vi "CreateVIActivationVIDesactivation.vi"(8 "error in (no error)":errorcluster, 11 "Menu in":refnum<class "VIActivation.lvclass">) -> (0 "error out":errorcluster, 3 "Menu out":refnum<class "VIActivation.lvclass">)   [LabVIEW 2021, in "VIActivation.lvlib" / "VIActivation.lvclass"]
uses:
  VIActivation.lvclass
  VIActivation.lvclass/VIActivation.ctl
  VIActivationEvents.ctl
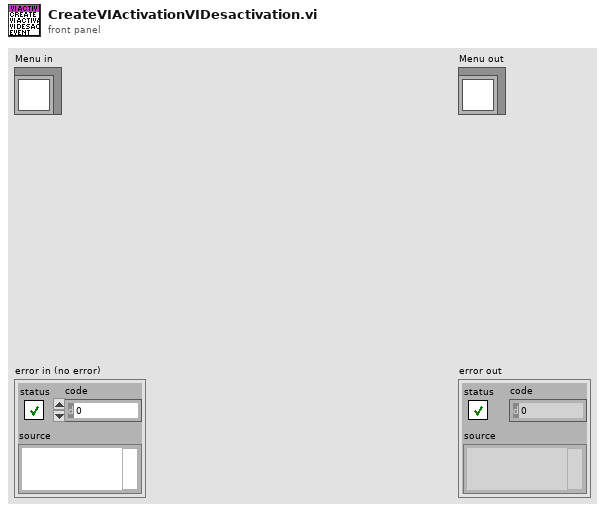
[diagram p1: front panel]
types:
  T1 = typedef "VIActivation.lvlib/VIActivation.lvclass/VIActivationEvents.ctl" = cluster{"AppRef":refnum<vi>, "VIName":string, "VIWindow":i32, "VIAppRef":refnum<vi>}
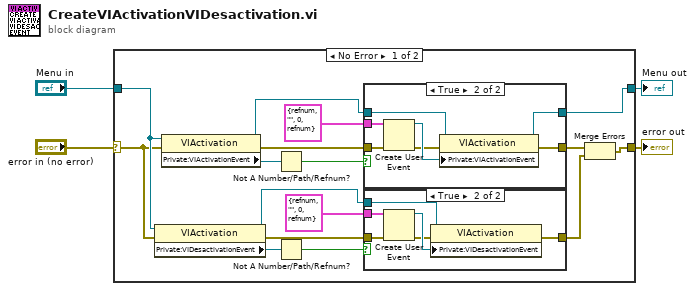
[diagram p0: block diagram]
diagram:
  n1 = case shown="No Error" "error in (no error)" {
    selector: "error in (no error)" -> [w6 w38]
    tunnel: [w11 w38] -> w3
    tunnel: [w20 w37] -> w1
    tunnel: "Menu in" -> [w9 w37]
    frame No Error {
      n2 = property class="VIActivation"(reference=w9, error in=w6) -> (reference out=w14:refnum<class "VIActivation.lvclass">, error out=w17:errorcluster, "Private:VIDesactivationEvent"=w13:refnum<user-event>)
      n3 = property class="VIActivation"(reference=w9, error in=w6) -> (reference out=w7:refnum<class "VIActivation.lvclass">, error out=w5:errorcluster, "Private:VIActivationEvent"=w8:refnum<user-event>)
      n4 = Not A Number/Path/Refnum?(number/path/refnum=w8) -> (NaN/Path/Refnum?=w19:bool)
      n5 = Not A Number/Path/Refnum?(number/path/refnum=w13) -> (NaN/Path/Refnum?=w15:bool)
      n6 = case shown="True" w19 {
        tunnel: w7 -> [w28 w36]
        tunnel: [w28 w35] -> w20
        tunnel: [w29 w34] -> w12
        tunnel: T1 {"AppRef"=refnum, "VIName"="", "VIWindow"=0, "VIAppRef"=refnum} ("VI Activation") -> [_ w33]
        tunnel: w5 -> [w29 w31]
        frame False {
        }
        frame True {
          n7 = Create User Event(user event datatype=w33, error in=w31) -> (user event=w32:refnum<user-event>, error out=w30:errorcluster)
          n8 = property class="VIActivation"(reference=w36, error in=w30, "Private:VIActivationEvent"=w32) -> (reference out=w35:refnum<class "VIActivation.lvclass">, error out=w34:errorcluster)
        }
      }
      n9 = case shown="True" w15 {
        tunnel: w14 -> [_ w27]
        tunnel: T1 {"AppRef"=refnum, "VIName"="", "VIWindow"=0, "VIAppRef"=refnum} ("VI Activation") -> [_ w26]
        tunnel: w17 -> [w21 w24]
        tunnel: [w21 w23] -> w10
        frame False {
        }
        frame True {
          n10 = Create User Event(user event datatype=w26, error in=w24) -> (user event=w25:refnum<user-event>, error out=w22:errorcluster)
          n11 = property class="VIActivation"(reference=w27, error in=w22, "Private:VIDesactivationEvent"=w25) -> (error out=w23:errorcluster)  [unwired: 1 out]
        }
      }
      n12 = Merge Errors(w12, w10) -> (w11:errorcluster)
    }
    frame Error {
    }
  }
  "error out" <- w3
  "Menu out" <- w1
